vi "TestConfig.vi"(8 "error in":errorcluster {"code" format="Error %.0f"}, 11 "MainFGV_data":T2={"TestDir"=path "", "TestName"="", "Simulation"=FALSE, "task"="", "data_file"=refnum, "burts_file"=refnum, "log_file"=refnum, "Rate"=0.0, "SamplesPerChannel"=0.0, "AcqQueue"=refnum, "StartTime"=timestamp(0 s since 1904-01-01), "config_channels"=[], "DAQmx Device"="", "delta_burst"=15.0}) -> (0 "error out":errorcluster {"code" format="Error %.0f"}, 3 "MainFGV_data out":T2={"TestDir"=path "", "TestName"="", "Simulation"=FALSE, "task"="", "data_file"=refnum, "burts_file"=refnum, "log_file"=refnum, "Rate"=0.0, "SamplesPerChannel"=0.0, "AcqQueue"=refnum, "StartTime"=timestamp(0 s since 1904-01-01), "config_channels"=[], "DAQmx Device"="", "delta_burst"=15.0})   [LabVIEW 2016]
uses:
  MainFGV_data.ctl
  config_board.ctl
  Log/log_mods.ctl
  Log/log_status.ctl
panel:
  in  "delta_burst":dbl=15.0 caption="Intervalo burts [min]"
  in  "rate":dbl=1000.0 caption="Taxa de aquisição [Hz]"
  in  "DAQmx Device":tag
  in  "config":T1[](array[typedef])
  in  "OK":bool
  in  "Cancelar":bool
  in  "OpenConfig":bool caption="Abrir\nconfiguração"
  in  "SaveConfig":bool caption="Salvar\nconfiguração"
  # "Configuração dos canais para o ensaio"
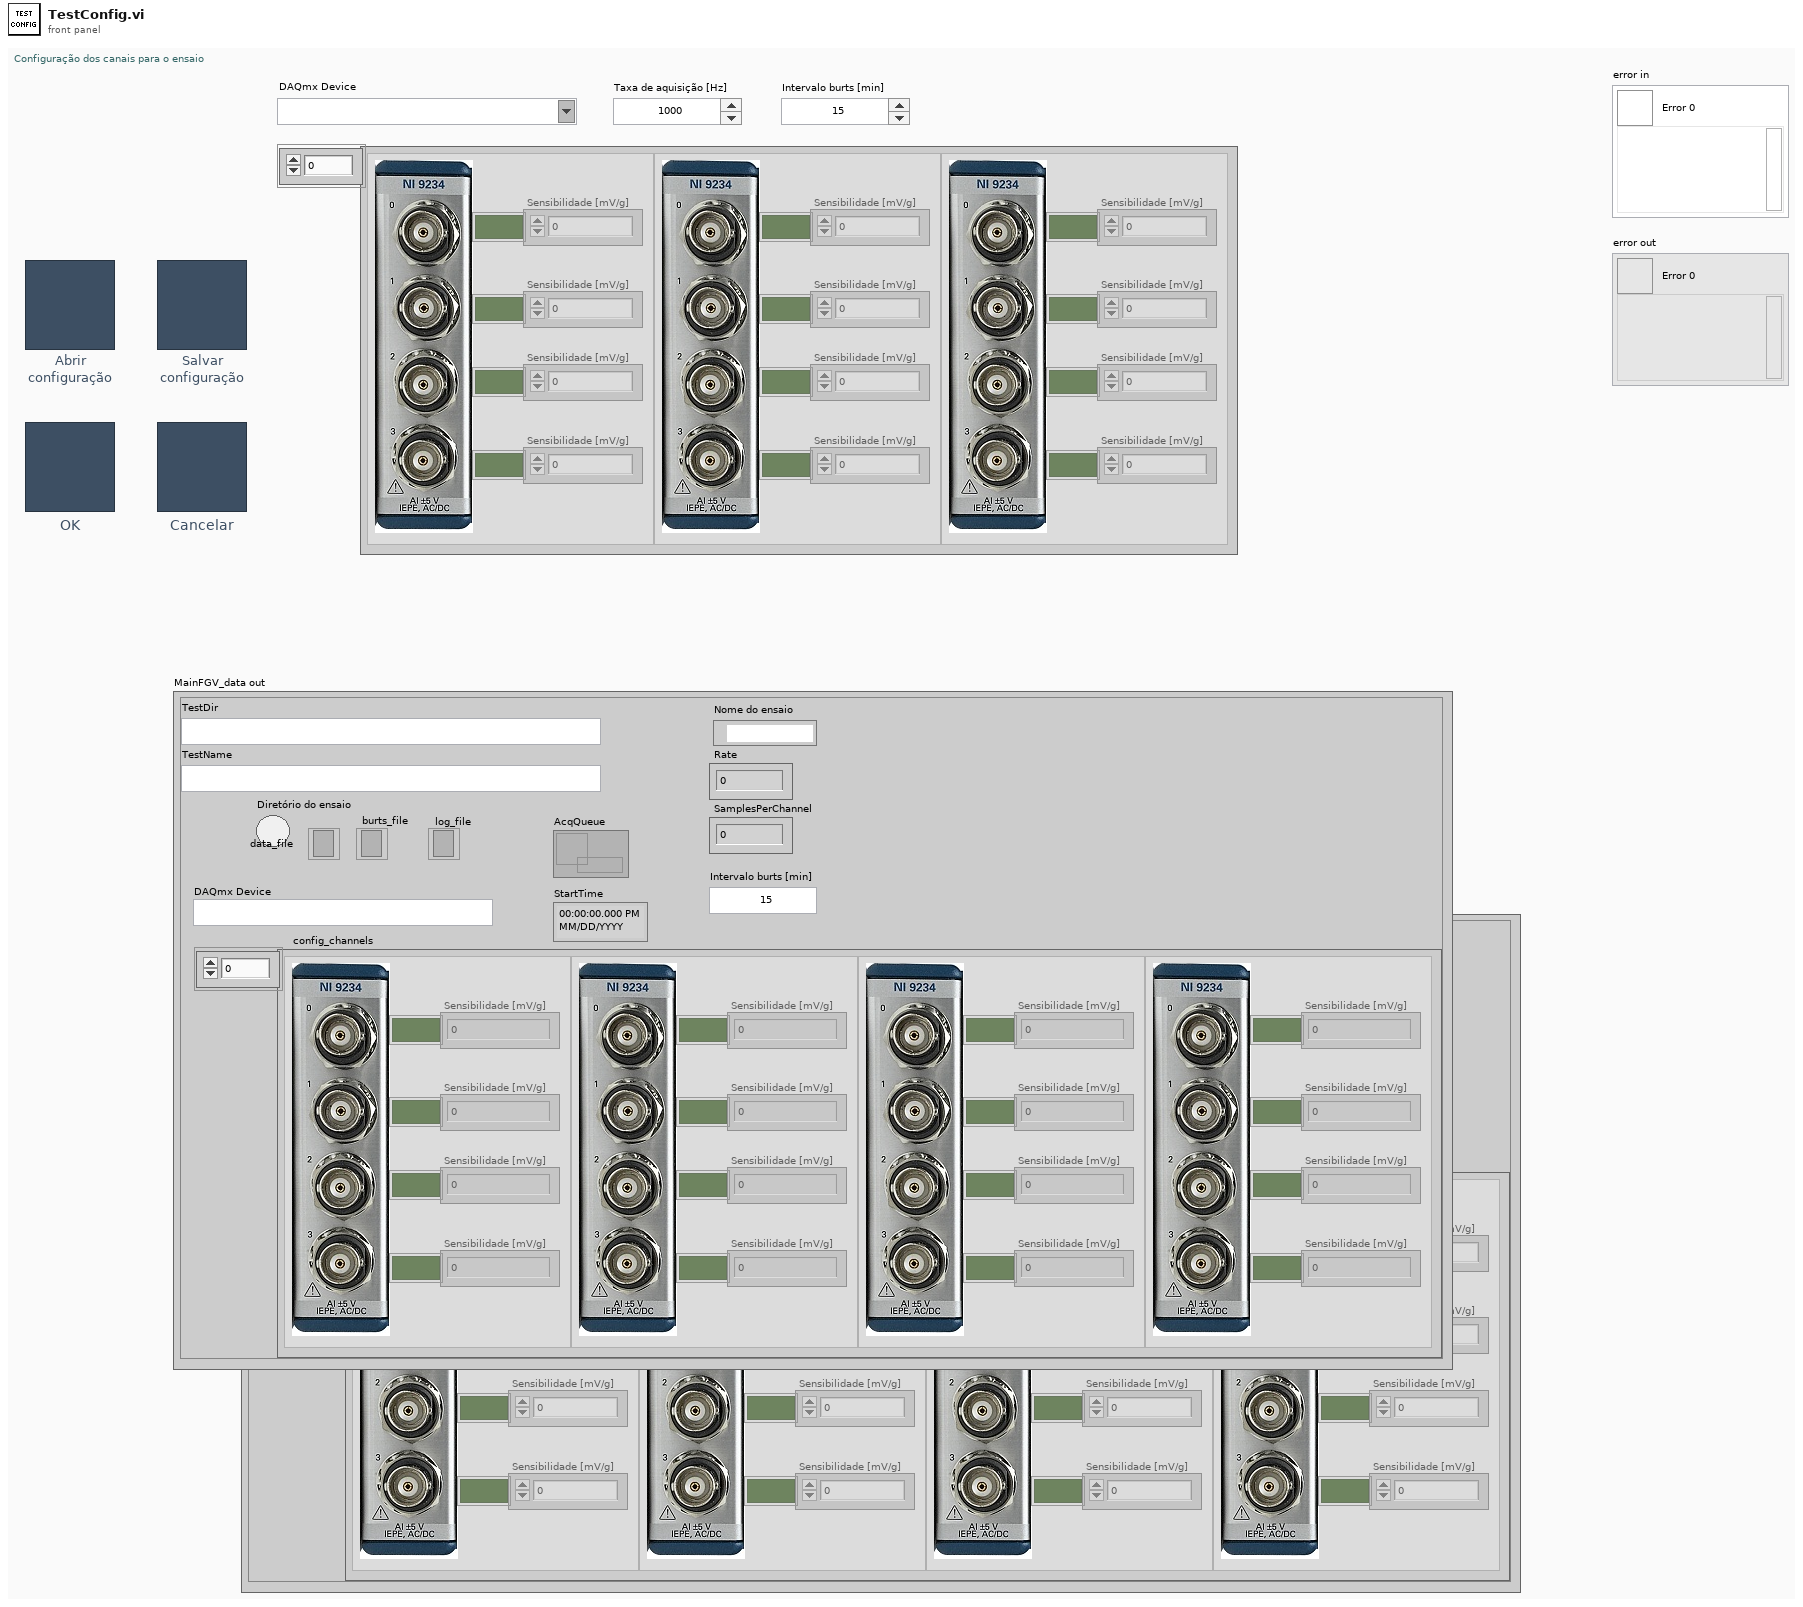
[diagram p1: front panel]
types:
  T1 = typedef "config_board.ctl" = cluster{"Sens0":dbl, "Active0":bool, "Sens1":dbl, "Active1":bool, "Sens2":dbl, "Active2":bool, "Sens3":dbl, "Active3":bool}
  T2 = typedef "MainFGV_data.ctl" = cluster{"TestDir":path, "TestName":string, "Simulation":bool, "task":refnum<k21>, "data_file":refnum<file>, "burts_file":refnum<file>, "log_file":refnum<file>, "Rate":dbl, "SamplesPerChannel":dbl, "AcqQueue":refnum<queue>, "StartTime":timestamp, "config_channels":T1[], "DAQmx Device":tag, "delta_burst":dbl}
  T3 = typedef "log_status.ctl" = enum16{"Init", "Ready", "Config", "Running", "Error", "End"}
  T4 = typedef "log_mods.ctl" = enum16{"Init", "LogFileRefnum", "SetStatus", "WriteAcel", "WriteToLog", "End"}
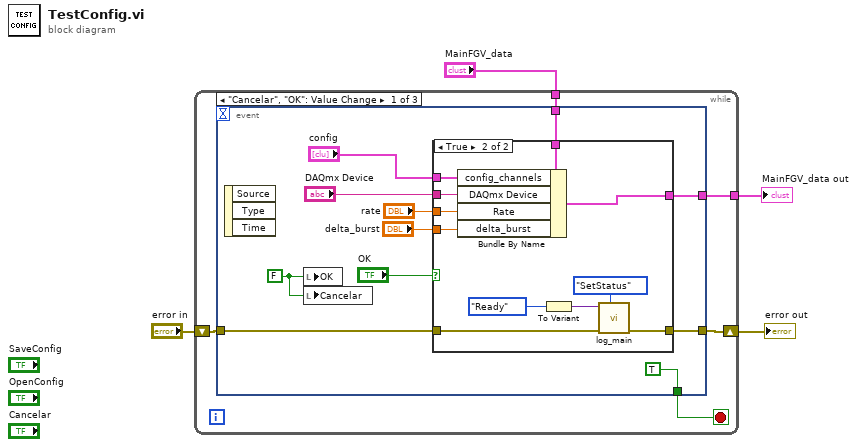
[diagram p0: block diagram]
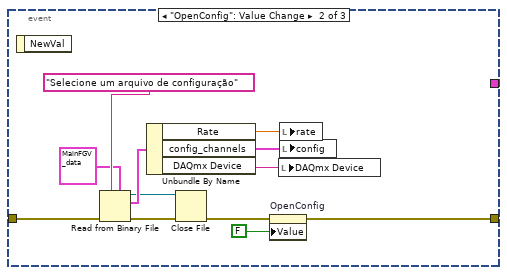
[diagram p3: hidden frame]
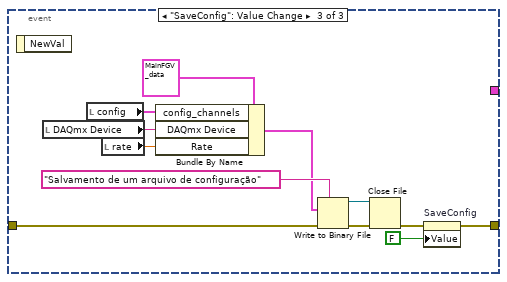
[diagram p4: hidden frame]
diagram:
  n1 = while {
    shift-right: [w7] -> w3
    shift-left: "error in" -> [w8]
    tunnel: "MainFGV_data" -> [w6]
    tunnel: [w5] -> w1
    stop <- w9 stop-if-true
    n2 = event shown="[0] \"Cancelar\", \"OK\": Value Change" {
      selector: _ -> [_ _ _]
      dyn-events: _ -> [_ _ _]
      timeout: _ -> [_ _ _]
      tunnel: [TRUE ("OK") _ _] -> w9
      tunnel: w8 -> [w15 w44 w53]
      tunnel: [w14 w35 w48] -> w7
      tunnel: w6 -> [w19 _ _]
      tunnel: [w18 _ _] -> w5
      event "Cancelar", "OK": Value Change {
        w17 = FALSE ("OK")
        n3 = event-data() -> ()  [unwired: 1 in, 3 out]
        n4 = local write "OK"(w17) -> ()
        n5 = local write "Cancelar"(w17) -> ()
        n6 = case shown="True" "OK" {
          tunnel: "DAQmx Device" -> [_ w33]
          tunnel: "config" -> [_ w32]
          tunnel: w19 -> [w22 w31]
          tunnel: [w22 w30] -> w18
          tunnel: w15 -> [w21 w26]
          tunnel: [w21 w25] -> w14
          tunnel: "rate" -> [_ w24]
          tunnel: "delta_burst" -> [_ w23]
          frame False {
          }
          frame True {
            n7 = Bundle By Name(cluster=w31, "config_channels"=w32, "DAQmx Device"=w33, "Rate"=w24, "delta_burst"=w23) -> (w30:T2)
            n8 = To Variant(anything=log_status."Ready" ("log_status")) -> (Variant=w27:variant)
            n9 = call "log_main.vi"("FGV_mods"=log_mods."SetStatus", "Error In"=w26, "DataIn"=w27) -> ("Error Out"=w25:errorcluster)  [unwired: 7 in, 1 out]
          }
        }
      }
      event "OpenConfig": Value Change {
        n10 = event-data() -> ()  [unwired: 1 in, 1 out]
        n11 = Read from Binary File(5:T2 {"TestDir"=path "C:/Users/l01481/Desktop/Teste_0", "TestName"="Teste", "Simulation"=TRUE, "task"="", "data_file"=refnum, "burts_file"=refnum, "log_file"=refnum, "Rate"=0.0, "SamplesPerChannel"=0.0, "AcqQueue"=refnum, "StartTime"=timestamp(0 s since 1904-01-01), "config_channels"=[], "DAQmx Device"="", "delta_burst"=15.0} ("MainFGV_data"), 7:"Selecione um arquivo de configuração" ("prompt (Open existing file)"), 8:w44) -> (0:w41:errorcluster, 2:w42:T2, 3:w40:refnum<file>)  [unwired: 3 in, 1 out]
        n12 = Unbundle By Name(w42) -> ("Rate"=w34:dbl, "config_channels"=w38:T1[], "DAQmx Device"=w39:tag)
        n13 = Close File(refnum=w40, error in=w41) -> (error out=w36:errorcluster)  [unwired: 1 out]
        n14 = property on="OpenConfig" class="Bool (strict)"(error in=w36, "Value"=FALSE ("SaveConfig")) -> (error out=w35:errorcluster)  [unwired: 1 in, 1 out]
        n15 = local write "DAQmx Device"(w39) -> ()
        n16 = local write "rate"(w34) -> ()
        n17 = local write "config"(w38) -> ()
      }
      event "SaveConfig": Value Change {
        n18 = event-data() -> ()  [unwired: 1 in, 1 out]
        n19 = local read "DAQmx Device"() -> (w55:tag)
        n20 = local read "config"() -> (w56:T1[])
        n21 = local read "rate"() -> (w46:dbl)
        n22 = Bundle By Name(cluster=T2 {"TestDir"=path "C:/Users/l01481/Desktop/Teste_0", "TestName"="Teste", "Simulation"=TRUE, "task"="", "data_file"=refnum, "burts_file"=refnum, "log_file"=refnum, "Rate"=0.0, "SamplesPerChannel"=0.0, "AcqQueue"=refnum, "StartTime"=timestamp(0 s since 1904-01-01), "config_channels"=[], "DAQmx Device"="", "delta_burst"=15.0} ("MainFGV_data"), "config_channels"=w56, "DAQmx Device"=w55, "Rate"=w46) -> (w50:T2)
        n23 = Write to Binary File(data=w50, error in=w53, 7:"Salvamento de um arquivo de configuração" ("prompt (Choose or enter file path)")) -> (refnum out=w51:refnum<file>, error out=w52:errorcluster)  [unwired: 3 in, 1 out]
        n24 = Close File(refnum=w51, error in=w52) -> (error out=w49:errorcluster)  [unwired: 1 out]
        n25 = property on="SaveConfig" class="Bool (strict)"(error in=w49, "Value"=FALSE ("SaveConfig")) -> (error out=w48:errorcluster)  [unwired: 1 in, 1 out]
      }
    }
  }
  "MainFGV_data out" <- w1
  "error out" <- w3
